vi "Split Cluster TD__ogtk.vi"(8 "error in (no error)":errorcluster, 10 "Type Descriptor":T1) -> (0 "error out":errorcluster, 2 "Type Descriptors":cluster{"Type Descriptor":T1}[](array[cluster]))   [LabVIEW 2020]
doc: "Splits the TD of a Cluster into its elements TDs."
uses:
  <userlib>/_OpenG.lib/lvdata/lvdata.llb/Type Descriptor__ogtk.ctl
panel:
  # "[OpenG VI Tags] ***Do Not Remove***"
  # "Split Cluster TD.vi\n\nSplits the TD of a Cluster into its elements TDs.\n\nPlease visit http://www.OpenG.org to learn about the\nOpen Source LabVIEW software movement.\n\nNOTICE -- YOU MUST LEAVE THIS NOTICE IN PLACE.  PER THE TERMS OF THE LICENSE BELOW, YOU MAY SUBLICENSE THIS SOFTWARE \nIN ANY WAY THAT DOES NOT CONFLICT WITH THIS LICENSE.\n\n### BSD License (http://www.opensource.org/licenses/bsd-license.php) Begin ###\n \nCopyright (c) 2002, Jean-Pierre Drolet <drolet_jp@hotmail.com>\nCopyright (c) 2002-2006, Jim Kring <jim@jimkring.com>\n\nAll rights reserved.\n\nRedistribution and use in source and binary forms, with or without modification, are permitted provided that the following conditions are met:\n\n    * Redistributions of source code must retain the above copyright notice, this list of conditions and the following disclaimer.\n    * Redistributions in binary form must reproduce the above copyright notice, this list of conditions and the following disclaimer in the \n       documentation and/or other materials provided with the distribution.\n    * Neither the name of SciWare, James Kring, Inc., nor the names of its contributors may be used to endorse or promote products derived \n       from this software without specific prior written permission.\n\nTHIS SOFTWARE IS PROVIDED BY THE COPYRIGHT HOLDERS AND CONTRIBUTORS \"AS IS\" AND ANY EXPRESS OR IMPLIED WARRANTIES, \nINCLUDING, BUT NOT LIMITED TO, THE IMPLIED WARRANTIES OF MERCHANTABILITY AND FITNESS FOR A PARTICULAR PURPOSE ARE \nDISCLAIMED. IN NO EVENT SHALL THE COPYRIGHT OWNER OR CONTRIBUTORS BE LIABLE FOR ANY DIRECT, INDIRECT, INCIDENTAL,\n SPECIAL, EXEMPLARY, OR CONSEQUENTIAL DAMAGES (INCLUDING, BUT NOT LIMITED TO, PROCUREMENT OF SUBSTITUTE GOODS OR \nSERVICES; LOSS OF USE, DATA, OR PROFITS; OR BUSINESS INTERRUPTION) HOWEVER CAUSED AND ON ANY THEORY OF LIABILITY, \nWHETHER IN CONTRACT, STRICT LIABILITY, OR TORT (INCLUDING NEGLIGENCE OR OTHERWISE) ARISING IN ANY WAY OUT OF THE USE \nOF THIS SOFTWARE, EVEN IF ADVISED OF THE POSSIBILITY OF SUCH DAMAGE.\n\n### BSD License End ###"
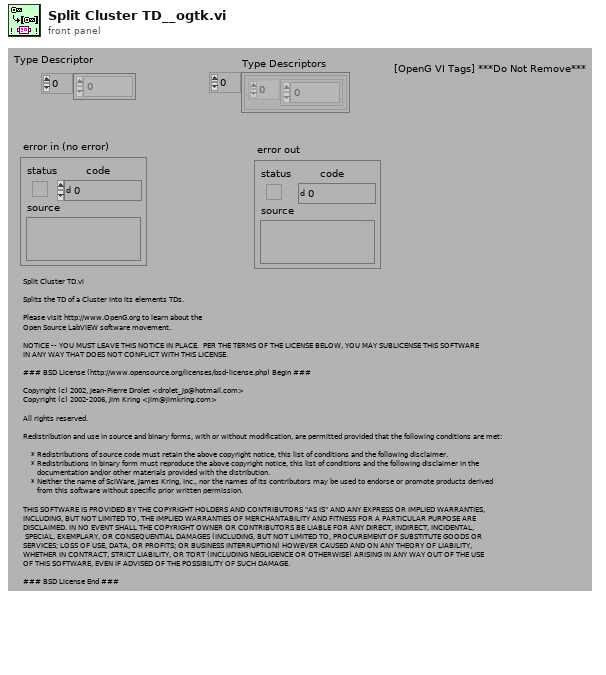
[diagram p1: front panel]
types:
  T1 = typedef "Type Descriptor__ogtk.ctl" = i16[]
  T2 = typedef "Type Descriptor Header__ogtk.ctl" = cluster{"length":u16, "private":u8, "type":T3, "# elements":u16}
  T3 = typedef "Type Descriptor Enumeration__ogtk.ctl" = enum8{"<Null>", "I8", "I16", "I32", "I64", "U8", "U16", "U32", "U64", "SGL", "DBL", "EXT", "CSG", "CDB", "CXT", "0x0F", "0x10", "0x11", "0x12", "0x13", "0x14", "Enum U8", "Enum U16", "Enum U32", "Enum U64", "SGL PQ", "DBL PQ", "EXT PQ", "CSG PQ", "CDB PQ", "CXT PQ", "0x1F", "0x20", "Boolean", "0x22", "0x23", "0x24", "0x25", "0x26", "0x27", "0x28", "0x29", "0x2A", "0x2B", "0x2C", "0x2D", "0x2E", "0x2F", "String", "0x31", "Path", "Pict", "0x34", "0x35", "0x36", "DAQ", "0x38", "0x39", "0x3A", "0x3B", "0x3C", "0x3D", "0x3E", "0x3F", "Array", "0x41", "0x42", "0x43", "0x44", "0x45", "0x46", "0x47", "0x48", "0x49", "0x4A", "0x4B", "0x4C", "0x4D", "0x4E", "0x4F", "Cluster", "0x51", "0x52", "Variant", "Waveform", "0x55", "0x56", "0x57", "0x58", "0x59", "0x5A", "0x5B", "0x5C", "0x5D", "0x5E", "Fixed Point", "0x60", "0x61", "0x62", "0x63", "0x64", "0x65", "0x66", "0x67", "0x68", "0x69", "0x6A", "0x6B", "0x6C", "0x6D", "0x6E", "0x6F", "Refnum", "0x71", "0x72", "Set Collection", "Map Collection"}
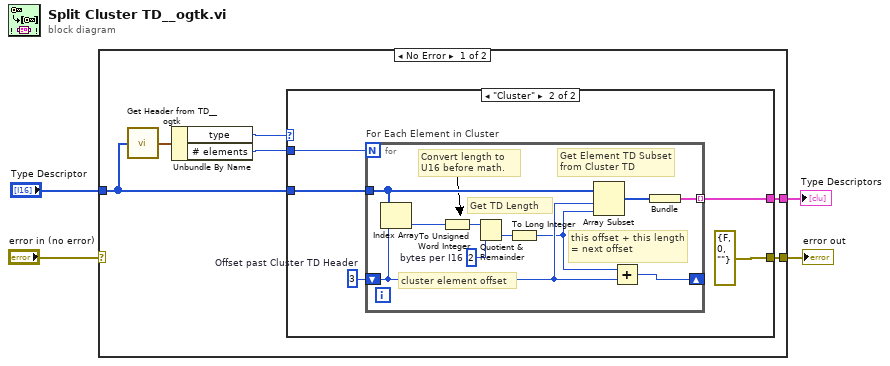
[diagram p0: block diagram]
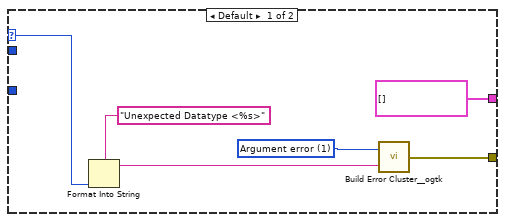
[diagram p2: hidden frame]
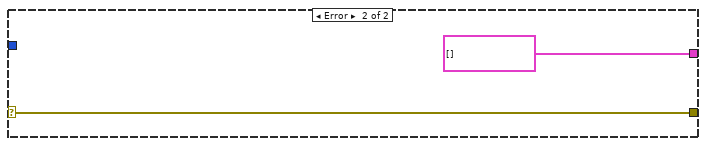
[diagram p3: hidden frame]
diagram:
  n1 = case shown="No Error" "error in (no error)" {
    selector: "error in (no error)" -> [_ w32]
    tunnel: [w8 cluster{i16[]}[] []] -> w3
    tunnel: [w7 w32] -> w2
    tunnel: "Type Descriptor" -> [w5 _]
    frame No Error {
      n2 = call <userlib>:"Get Header from TD__ogtk.vi"("Type Descriptor"=w5) -> ("Type Descriptor Header"=w6:T2)
      n3 = Unbundle By Name(w6) -> ("type"=w10:T3, "# elements"=w9:u16)
      n4 = case shown="\"Cluster\"" w10 {
        selector: w10 -> [w11 _]
        tunnel: w9 -> [_ w20]
        tunnel: w5 -> [_ w19]
        tunnel: [cluster{i16[]}[] [] w18] -> w8
        tunnel: [w15 errorcluster {"status"=FALSE, "code"=0, "source"=""} ("error out")] -> w7
        frame Default {
          w16 = 1 items=["No error", "Argument error", "Memory is full", "Out of zone", "End of file", "File already open", "Generic file I/O error", "File not found", "File permission error", "Disk is full", "Duplicate path", "Too many files open", "System feature not enabled", "Resource file not found", "Cannot add resource", "Resource not found", "Image not found", "Image memory error", "Pen does not exist", "Config type invalid", "Config token not found", "Config parse error", "Config memory error", "Bad external code format", "Bad external code offset", "External code not present", "Null window", "Destroy window error", "Null menu", "Print aborted", "Bad print record", "Print driver error", "Windows error during printing", "Memory error during printing", "Print dialog error", "Generic print error", "Invalid device refnum", "Device not found", "Device parameter error", "Device unit error", "Cannot open device", "Device call aborted", "Generic error", "Cancelled by user", "Object ID too low", "Object ID too high", "Object not in heap", "Unknown heap", "Unknown object (invalid DefProc)", "Unknown object (DefProc not in table)", "Message out of range", "Invalid (null) method", "Unknown message", "Manager call not supported", "Bad address", "Network operation in progress", "Network operation timed out", "Connection is busy", "Network attribute not supported", "Network error", "Address in use", "System out of memory", "Connection aborted", "Connection refused", "Not connected", "Already connected", "Connection closed", "Initialization error (interapplication manager)", "Bad occurrence", "Wait on unbound occurrence handler", "Occurrence queue overflow", "Datalog type conflict", "Unused", "Unrecognized type (interapplication manager)", "Memory corrupt", "Failed to make temporary DLL", "Old CIN version", "Drag socket not found", "Failed to load drop-object", "Failed to register OLE object", "Failed to release OLE object", "Format specifier type mismatch", "Unknown format specifier", "Too few format specifiers", "Too many format specifiers", "Scan failed", "Newer CIN version", "Error converting to variant", "Runtime menu error", "Password tampered", "Variant attribute not found", "Incompatible variant data type", "Event data is not available", "Event Store is not present", "Occurrence is not found", "Event Queue is not created", "Event info is not available", "Refnum passed is NULL", "Error retrieving Class GUID", "Error retrieving CoClass GUID", "Error retrieving TypeLib GUID.", "Bad built application magic bytes.", "Specific driver is different from the specific driver associated with the Logical Name.", "There is no session opened to the class driver.", "Max Error", "MAX - Error with config objects", "MAX - Error loading configuration", "MAX - Group not supported"]
          n5 = Format Into String(format string="Unexpected Datatype <%s>" ("Format String"), w11) -> (resulting string=w12:string)  [unwired: 2 in, 1 out]
          n6 = call <userlib>:"Build Error Cluster__ogtk.vi"("String to Prepend to source (\"\")"=w12, "code"=w16) -> ("error out"=w15:errorcluster)
        }
        frame "Cluster" {
          w21 = 3  # Offset past Cluster TD Header
          n7 = for "For Each Element in Cluster" {
            N: w20 -> [_]
            shift-right: [w29] -> _
            shift-left: w21 -> [w28]
            tunnel: w19 -> [w30]
            tunnel: [w24] -> w18 mode=indexing
            w25 = u16 2  # bytes per I16
            # "Get TD Length"
            # "this offset + this length = next offset"
            # "cluster element offset"
            # "Get Element TD Subset from Cluster TD"
            # "Convert length to U16 before math."
            n8 = Index Array(array=w30, index=w28) -> (element=w26:i16)
            n9 = To Unsigned Word Integer(number=w26) -> (unsigned 16bit integer=w23:u16)
            n10 = Quotient & Remainder(x=w23, y=w25) -> (floor(x/y)=w27:u16)  [unwired: 1 out]
            n11 = To Long Integer(number=w27) -> (32bit integer=w22:i32)
            n12 = Array Subset(array=w30, index=w28, length=w22) -> (w31:T1)
            n13 = Add(x=w22, y=w28) -> (x+y=w29:i32)
            n14 = Bundle(w31) -> (w24:cluster{T1})  [unwired: 1 in]
          }
        }
      }
    }
    frame Error {
    }
  }
  "error out" <- w2
  "Type Descriptors" <- w3
